vi "SetLevel.vi"(8 "error in (no error)":errorcluster, 10 "level":dbl, 11 "SpecA_MXA in":refnum<class "SpecA_MXA.lvclass">) -> (0 "error out":errorcluster, 3 "SpecA_MXA out":refnum<class "SpecA_MXA.lvclass">)   [LabVIEW 2014, in "SpecA_MXA.lvclass"]
uses:
  SpecA_MXA.lvclass
  SpecA_MXA.lvclass/SpecA_MXA.ctl
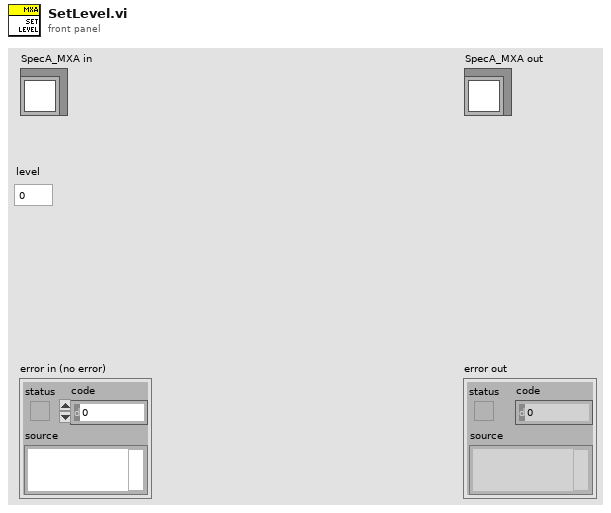
[diagram p1: front panel]
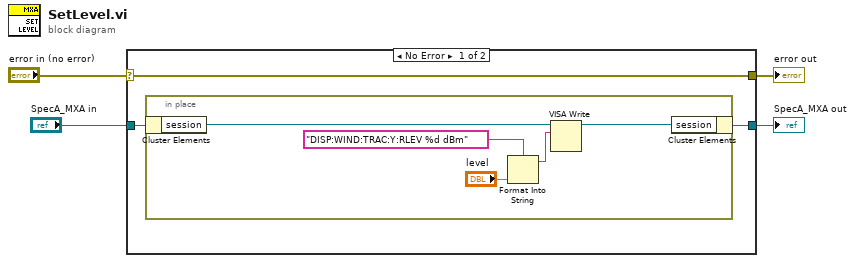
[diagram p0: block diagram]
diagram:
  n1 = case shown="No Error" "error in (no error)" {
    selector: "error in (no error)" -> [w7 w14]
    tunnel: [w7 w14] -> w3
    tunnel: "SpecA_MXA in" -> [w6 w13]
    tunnel: [w5 w13] -> w1
    frame No Error {
      n2 = in-place {
        n3 = in-place-cluster #1(w6) -> ("session"=w9:refnum<visa-resource-name>)
        n4 = Format Into String(format string="DISP:WIND:TRAC:Y:RLEV %d dBm", "level") -> (resulting string=w11:string)  [unwired: 2 in, 1 out]
        n5 = VISA Write(VISA resource name=w9, write buffer=w11) -> (VISA resource name out=w8:refnum<visa-resource-name>)  [unwired: 1 in, 2 out]
        n6 = in-place-cluster #1("session"=w8) -> (w5:refnum<class "SpecA_MXA.lvclass">)
      }
    }
    frame Error {
    }
  }
  "error out" <- w3
  "SpecA_MXA out" <- w1
